vi "Read Total Counts.vi"(8 "error in (no error)":errorcluster, 11 "Analyze Results Total Counts in":refnum<class "Analyze Results Total Counts.lvclass">) -> (0 "error out":errorcluster, 2 "Total Counts":dbl, 3 "Analyze Results Total Counts out":refnum<class "Analyze Results Total Counts.lvclass">)   [LabVIEW 2014, in "Analyze Results Total Counts.lvclass"]
uses:
  Analyze Results Total Counts.lvclass
  Analyze Results Total Counts.lvclass/Analyze Results Total Counts.ctl
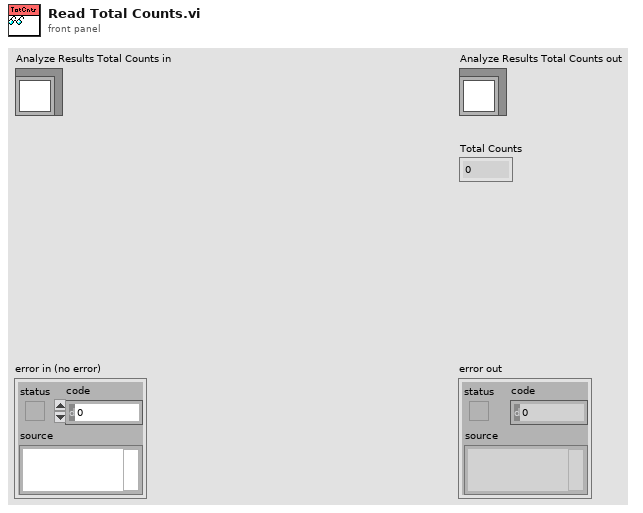
[diagram p1: front panel]
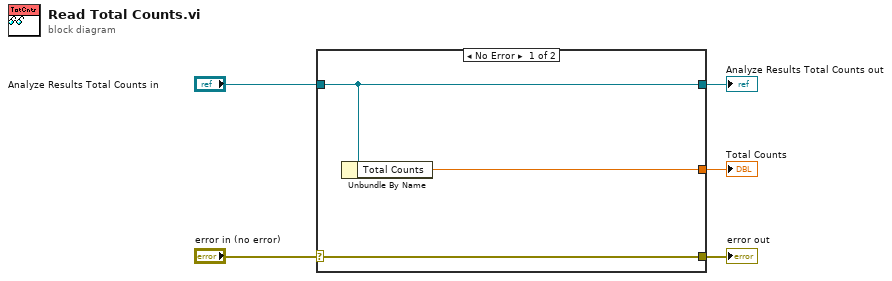
[diagram p0: block diagram]
diagram:
  n1 = case shown="No Error" "error in (no error)" {
    selector: "error in (no error)" -> [w8 w9]
    tunnel: [w8 w9] -> w4
    tunnel: [w7 w10] -> w2
    tunnel: "Analyze Results Total Counts in" -> [w7 w10]
    tunnel: [w6 _] -> w1
    frame No Error {
      n2 = Unbundle By Name(w7) -> ("Total Counts"=w6:dbl)
    }
    frame Error {
    }
  }
  "error out" <- w4
  "Analyze Results Total Counts out" <- w2
  "Total Counts" <- w1
